vi "read_P_Dop.vi"(12 "P_Dop Flow 2":dbl, 14 "P_Dop Flow 1":dbl) -> (0 "N/P Dopant DA Switch":bool, 1 "P_Dop Active":bool, 2 "P_Dop Bubbler":bool, 3 "P_Dop H2 Dilute":bool, 4 "P_Dop Gas Source":bool, 5 "P_Dop Run":bool, 6 "P_Dop Remote":bool, 10 "P_Dop Flow 3":dbl)   [LabVIEW 2011]
panel:
  out "Actual P Dopant Flow Rate 4":dbl
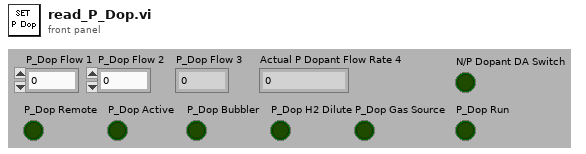
[diagram p1: front panel]
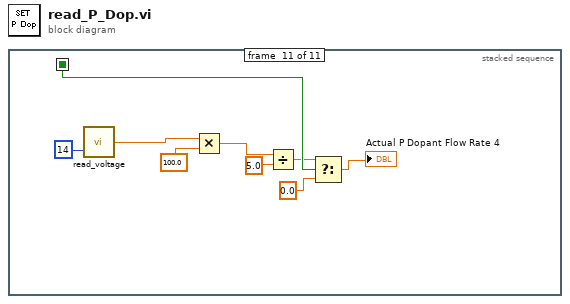
[diagram p0: block diagram]
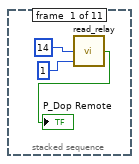
[diagram p2: hidden frame]
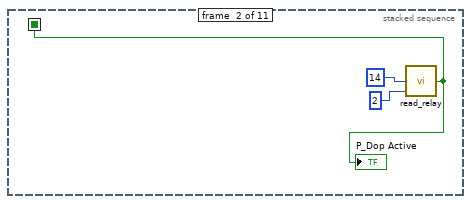
[diagram p3: hidden frame]
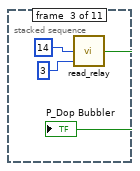
[diagram p4: hidden frame]
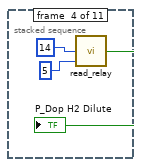
[diagram p5: hidden frame]
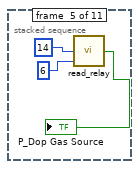
[diagram p6: hidden frame]
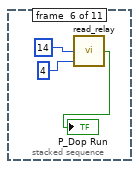
[diagram p7: hidden frame]
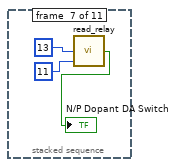
[diagram p8: hidden frame]
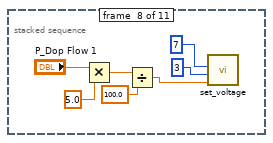
[diagram p9: hidden frame]
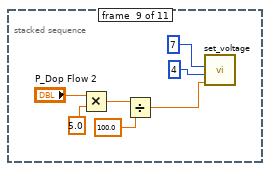
[diagram p10: hidden frame]
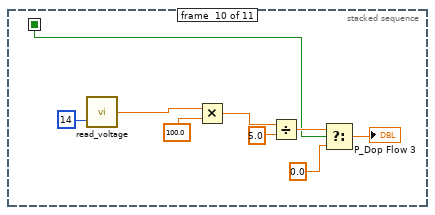
[diagram p11: hidden frame]
diagram:
  n1 = stacked-sequence {
    seq-local: [_ w4 _ _ _ _ _ _ _ _ _] -> [_ _ _ _ _ _ _ _ _ w38 w48]
    frame #0 {
      n2 = call "read_relay.vi"("Relay"=1, "Slot"=14) -> ("Relay Status"=→"P_Dop Remote":bool)  [unwired: 1 out]
    }
    frame #1 {
      n3 = call "read_relay.vi"("Relay"=2, "Slot"=14) -> ("Relay Status"=w4:bool)  [unwired: 1 out]
      "P_Dop Active" <- w4
    }
    frame #2 {
      n4 = call "read_relay.vi"("Relay"=3, "Slot"=14) -> ("Relay Status"=→"P_Dop Bubbler":bool)  [unwired: 1 out]
    }
    frame #3 {
      n5 = call "read_relay.vi"("Relay"=5, "Slot"=14) -> ("Relay Status"=→"P_Dop H2 Dilute":bool)  [unwired: 1 out]
    }
    frame #4 {
      n6 = call "read_relay.vi"("Relay"=6, "Slot"=14) -> ("Relay Status"=→"P_Dop Gas Source":bool)  [unwired: 1 out]
    }
    frame #5 {
      n7 = call "read_relay.vi"("Relay"=4, "Slot"=14) -> ("Relay Status"=→"P_Dop Run":bool)  [unwired: 1 out]
    }
    frame #6 {
      n8 = call "read_relay.vi"("Relay"=11, "Slot"=13) -> ("Relay Status"=→"N/P Dopant DA Switch":bool)  [unwired: 1 out]
    }
    frame #7 {
      n9 = Multiply(x="P_Dop Flow 1", y=5.0) -> (x*y=w25:dbl)
      n10 = Divide(x=w25, y=100.0) -> (x/y=w27:dbl)
      n11 = call "set_voltage.vi"("Voltage"=w27, "Channel"=3, "Slot"=7) -> ()  [unwired: 1 in, 1 out]
    }
    frame #8 {
      n12 = Multiply(x="P_Dop Flow 2", y=5.0) -> (x*y=w29:dbl)
      n13 = Divide(x=w29, y=100.0) -> (x/y=w34:dbl)
      n14 = call "set_voltage.vi"("Voltage"=w34, "Channel"=4, "Slot"=7) -> ()  [unwired: 1 in, 1 out]
    }
    frame #9 {
      n15 = call "read_voltage.vi"("Channel"=14) -> ("Voltage"=w40:dbl)  [unwired: 1 in]
      n16 = Multiply(x=w40, y=100.0) -> (x*y=w42:dbl)
      n17 = Divide(x=w42, y=5.0) -> (x/y=w39:dbl)
      n18 = Select(t=w39, s=w38, f=0.0) -> (s? t:f=→"P_Dop Flow 3":dbl)
    }
    frame #10 {
      n19 = call "read_voltage.vi"("Channel"=14) -> ("Voltage"=w53:dbl)  [unwired: 1 in]
      n20 = Multiply(x=w53, y=100.0) -> (x*y=w51:dbl)
      n21 = Divide(x=w51, y=5.0) -> (x/y=w47:dbl)
      n22 = Select(t=w47, s=w48, f=0.0) -> (s? t:f=→"Actual P Dopant Flow Rate 4":dbl)
    }
  }
